vi "Get Result.vi"(8 "error in (no error)":errorcluster, 11 "IV in":refnum<class "IV.lvclass">) -> (0 "error out":errorcluster, 1 "Lockin result":refnum<class "Acquired Result.lvclass">, 2 "Curent source result":refnum<class "Acquired Result.lvclass">, 3 "IV out":refnum<class "IV.lvclass">, 4 "Temperature result":refnum<class "Acquired Result.lvclass">)   [LabVIEW 2021, in "IV.lvclass"]
uses:
  IV.lvclass
  Libraries/Instruments/Results/Acquired Result/Acquired Result.lvclass
  Libraries/Instruments/Instrument Driver/Instrument Driver.lvclass
  Libraries/File/File Class/File.lvclass
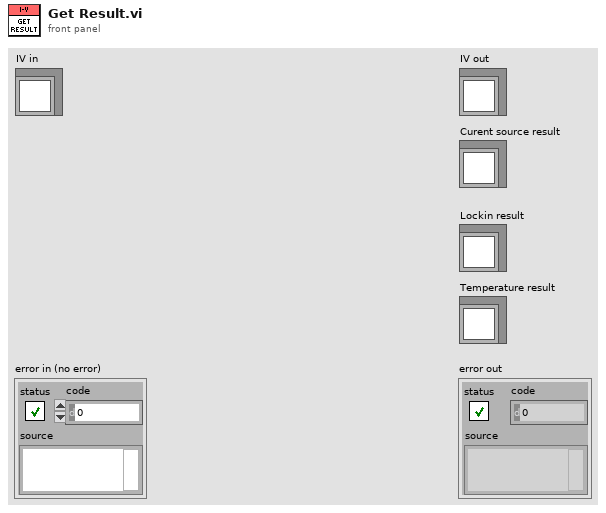
[diagram p1: front panel]
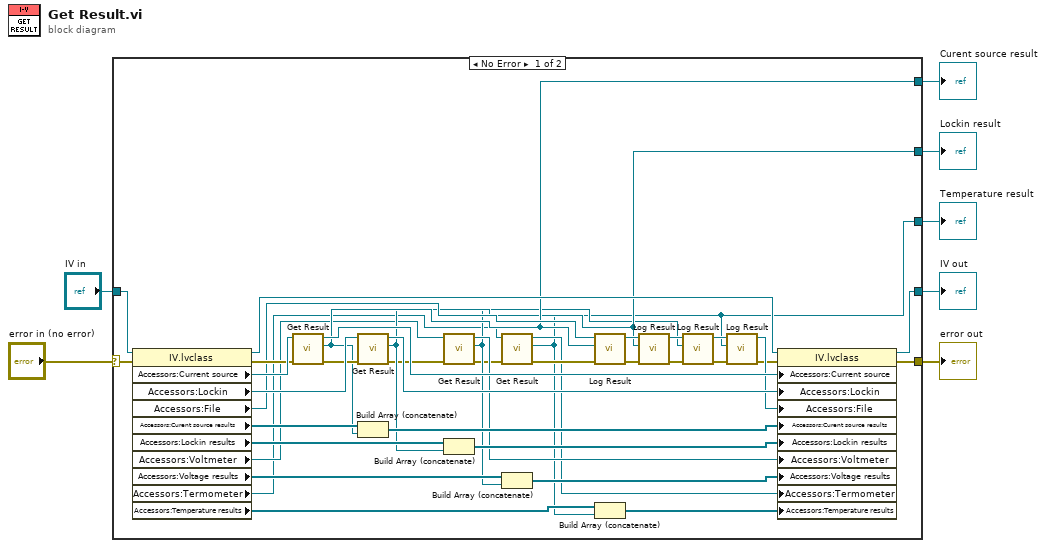
[diagram p0: block diagram]
diagram:
  n1 = case shown="No Error" "error in (no error)" {
    selector: "error in (no error)" -> [w46 w48]
    tunnel: [w44 w48] -> w6
    tunnel: [w42 w47] -> w4
    tunnel: "IV in" -> [w45 w47]
    tunnel: [w28 _] -> w3
    tunnel: [w30 _] -> w2
    tunnel: [w8 _] -> w1
    frame No Error {
      n2 = property class="IV.lvclass"(reference=w45, error in=w46) -> (reference out=w43:refnum<class "IV.lvclass">, error out=w36:errorcluster, "Accessors:Current source "=w39:refnum<class "Instrument Driver.lvclass">, "Accessors:Lockin"=w41:refnum<class "Instrument Driver.lvclass">, "Accessors:File"=w35:refnum<class "File.lvclass">, "Accessors:Curent source results"=w32:refnum<class "Acquired Result.lvclass">[], "Accessors:Lockin results"=w29:refnum<class "Acquired Result.lvclass">[], "Accessors:Voltmeter"=w26:refnum<class "Instrument Driver.lvclass">, "Accessors:Voltage results"=w24:refnum<class "Acquired Result.lvclass">[], "Accessors:Termometer"=w18:refnum<class "Instrument Driver.lvclass">, "Accessors:Temperature results"=w15:refnum<class "Acquired Result.lvclass">[])
      n3 = call-dynamic "Get Result.vi"("error in (no error)"=w36, "Instrument Driver in"=w39) -> ("error out"=w37:errorcluster, "Result"=w30:refnum<class "Acquired Result.lvclass">, "Instrument Driver out"=w38:refnum<class "Instrument Driver.lvclass">)  [unwired: 7 in]
      n4 = call-dynamic "Get Result.vi"("error in (no error)"=w37, "Instrument Driver in"=w41) -> ("error out"=w25:errorcluster, "Result"=w28:refnum<class "Acquired Result.lvclass">, "Instrument Driver out"=w40:refnum<class "Instrument Driver.lvclass">)  [unwired: 7 in]
      n5 = Build Array (concatenate)(w32, w30) -> (w31:refnum<class "Acquired Result.lvclass">[])
      n6 = call-dynamic "Get Result.vi"("error in (no error)"=w25, "Instrument Driver in"=w26) -> ("error out"=w17:errorcluster, "Result"=w19:refnum<class "Acquired Result.lvclass">, "Instrument Driver out"=w22:refnum<class "Instrument Driver.lvclass">)  [unwired: 7 in]
      n7 = Build Array (concatenate)(w29, w28) -> (w27:refnum<class "Acquired Result.lvclass">[])
      n8 = call-dynamic "Get Result.vi"("error in (no error)"=w17, "Instrument Driver in"=w18) -> ("error out"=w16:errorcluster, "Result"=w8:refnum<class "Acquired Result.lvclass">, "Instrument Driver out"=w14:refnum<class "Instrument Driver.lvclass">)  [unwired: 7 in]
      n9 = Build Array (concatenate)(w24, w19) -> (w23:refnum<class "Acquired Result.lvclass">[])
      n10 = call-dynamic "Log Result.vi"("error in (no error)"=w16, "Result"=w30, "File in"=w35) -> ("error out"=w34:errorcluster, "File out"=w33:refnum<class "File.lvclass">)  [unwired: 7 in]
      n11 = Build Array (concatenate)(w15, w8) -> (w13:refnum<class "Acquired Result.lvclass">[])
      n12 = call-dynamic "Log Result.vi"("error in (no error)"=w34, "Result"=w28, "File in"=w33) -> ("error out"=w20:errorcluster, "File out"=w21:refnum<class "File.lvclass">)  [unwired: 7 in]
      n13 = call-dynamic "Log Result.vi"("error in (no error)"=w20, "Result"=w19, "File in"=w21) -> ("error out"=w10:errorcluster, "File out"=w12:refnum<class "File.lvclass">)  [unwired: 7 in]
      n14 = call-dynamic "Log Result.vi"("error in (no error)"=w10, "Result"=w8, "File in"=w12) -> ("error out"=w9:errorcluster, "File out"=w11:refnum<class "File.lvclass">)  [unwired: 7 in]
      n15 = property class="IV.lvclass"(reference=w43, error in=w9, "Accessors:Current source "=w38, "Accessors:Lockin"=w40, "Accessors:File"=w11, "Accessors:Curent source results"=w31, "Accessors:Lockin results"=w27, "Accessors:Voltmeter"=w22, "Accessors:Voltage results"=w23, "Accessors:Termometer"=w14, "Accessors:Temperature results"=w13) -> (reference out=w42:refnum<class "IV.lvclass">, error out=w44:errorcluster)
    }
    frame Error {
    }
  }
  "error out" <- w6
  "IV out" <- w4
  "Lockin result" <- w3
  "Curent source result" <- w2
  "Temperature result" <- w1
